vi "SeCrTs-DO Data FGV.vi"(0 "DO Values In":bool[](array[boolean]), 1 "Option":T1(ring)=enum."Start Pattern Mode", 5 "DO Channel Names":string[](array[string]), 9 "Time Stamp In":timestamp, 11 "error in (no error)":errorcluster, 12 "DO Pattern Values In":bool[][](array[boolean])) -> (3 "Expected Completed Time (Pattern)":timestamp, 4 "DO Values Out":bool[](array[boolean]), 6 "All data out":waveform(dbl)[](array[waveform]), 8 "DO Channel Names Out":string[](array[string]), 10 "DO Waveform Out":digitalwaveform[](array[waveform]), 14 "Time Stamp Out":timestamp, 15 "error out":errorcluster)   [LabVIEW 2022 SP3]
uses:
  RT Controls/SeCrTs-FGV Read write.ctl
  <vilib>/Waveform/DTblOps.llb/DTbl Boolean Array to Digital.vi
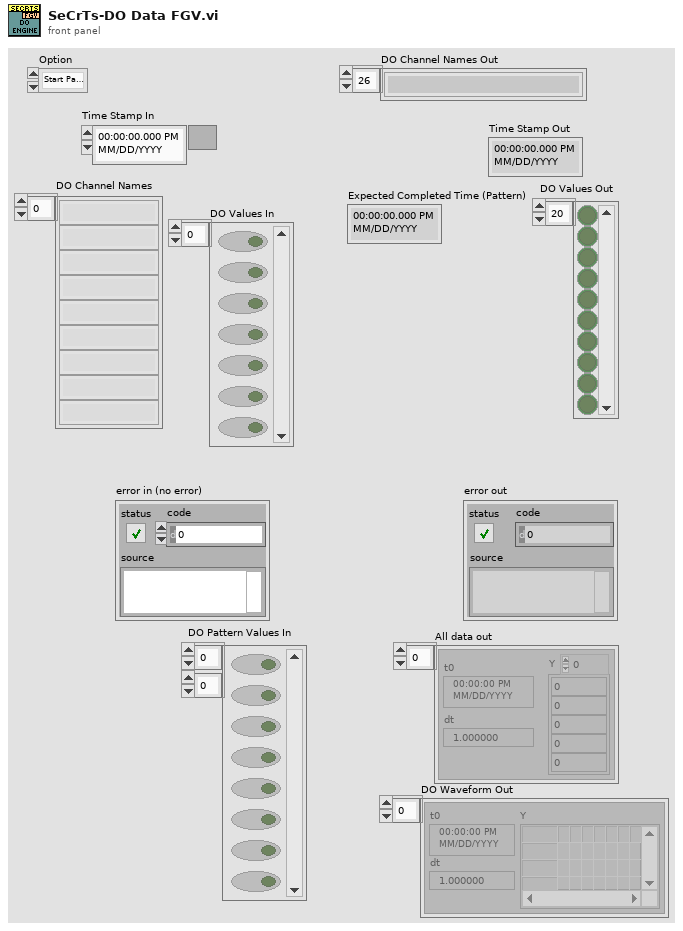
[diagram p1: front panel]
types:
  T1 = enum16{"Init", "Read", "Write 'All'", "Write 'n'", "Write Safe Value", "Write Start Time", "Overwrite Pattern", "Overwrite Pattern with Start", "Append Pattern", "Start Pattern Mode", "Abort Pattern Mode", "Read 1"}
  T2 = typedef "SeCrTs-FGV Read write.ctl" = enum16{"Write", "Read"}
  T3 = cluster{"Samples to Read":i32, "Pattern Mode?":bool, "dt(sec)":dbl, "DO Init Time (Samples)":i32, "dt per Read/Write":dbl, "Write Pointer":i32, "Pattern Size":i32, "Loop Rate (mSec)":i32, "Buffer Size (Samples)":i32, "Sampling rate":dbl, "Max DO Delay Time (samples)":dbl, "Min DO Delay Time (samples)":dbl, "Queue Size":i32, "DO Init Sample Duration (Sec)":dbl}
  T4 = cluster{"Pattern Size":i32, "Write Pointer":i32, "DO Channel Names":string[], "Pattern Mode?":bool, "DO Safe Waveform":waveform(dbl)[], "DO Safe Digital Waveform":digitalwaveform[], "DO Safe Values In":bool[], "dt per Read/Write":dbl}
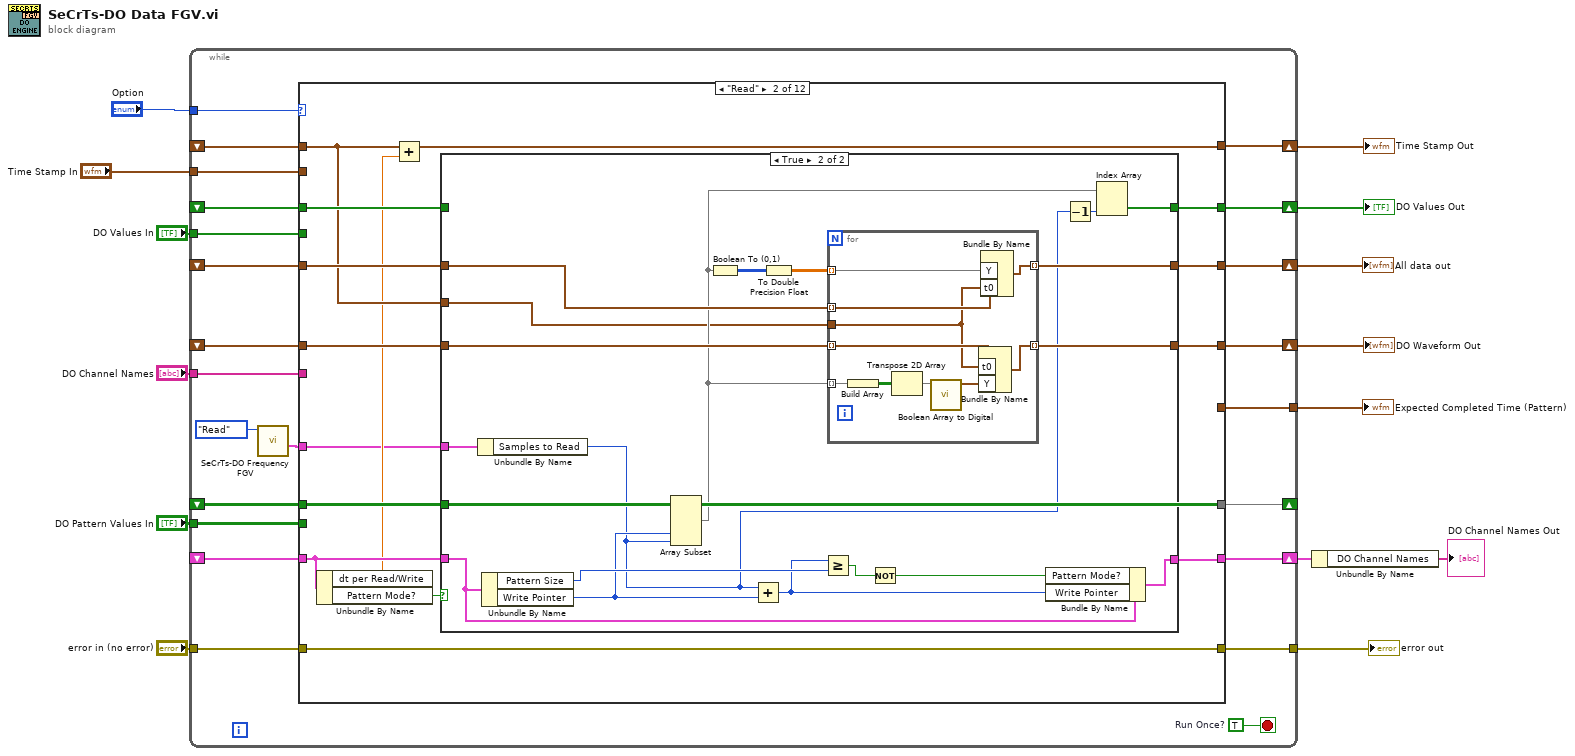
[diagram p0: block diagram]
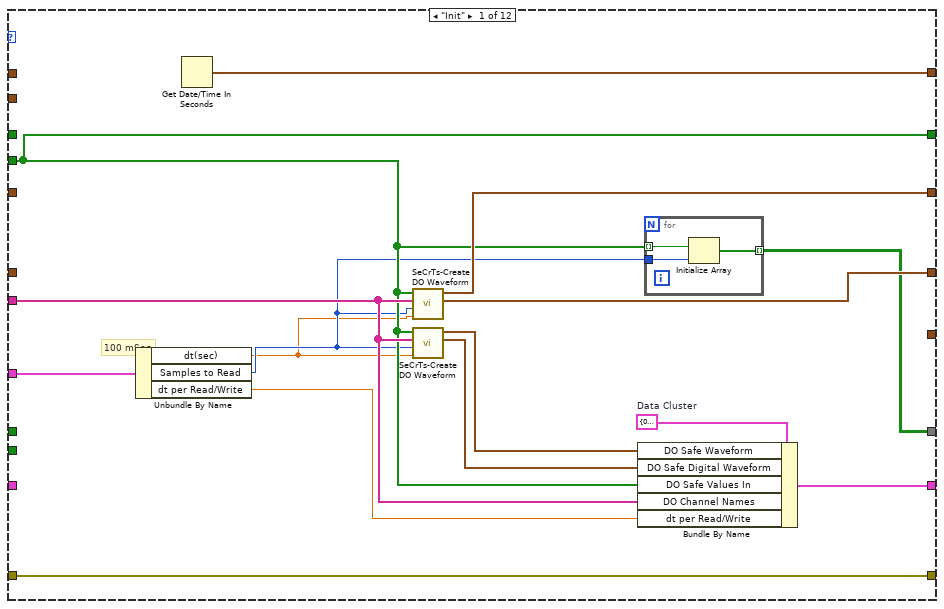
[diagram p2: hidden frame]
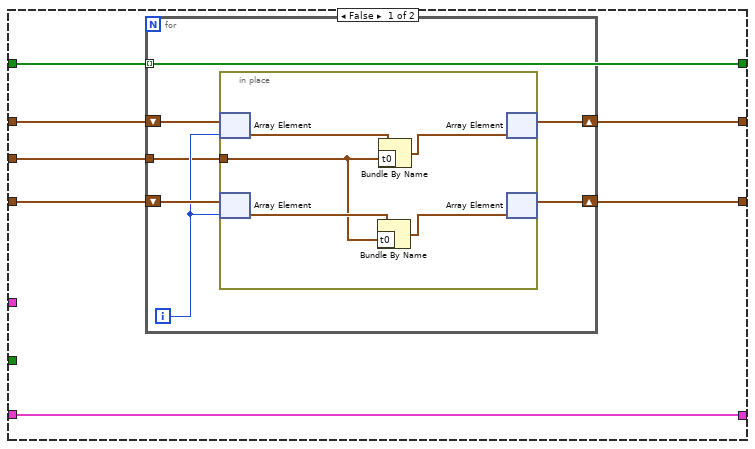
[diagram p3: hidden frame]
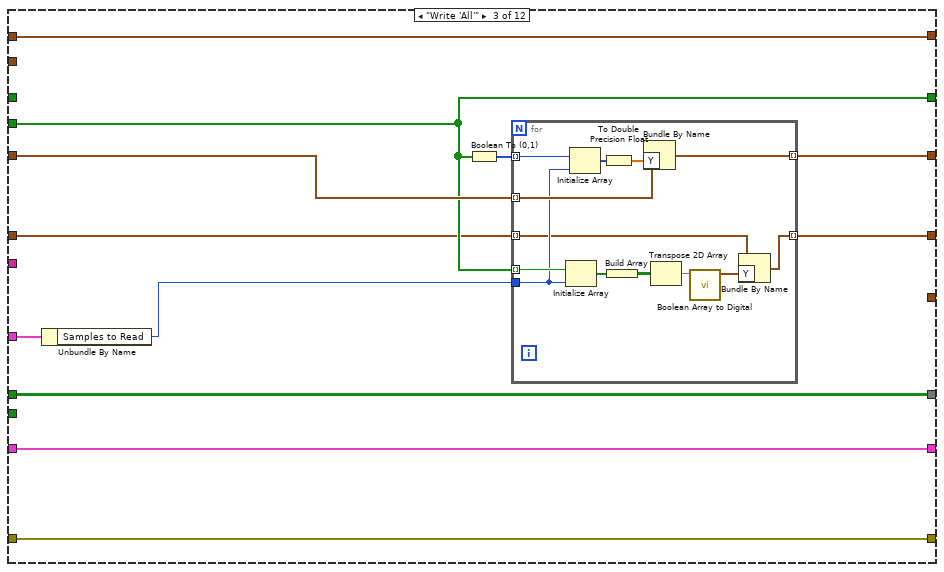
[diagram p4: hidden frame]
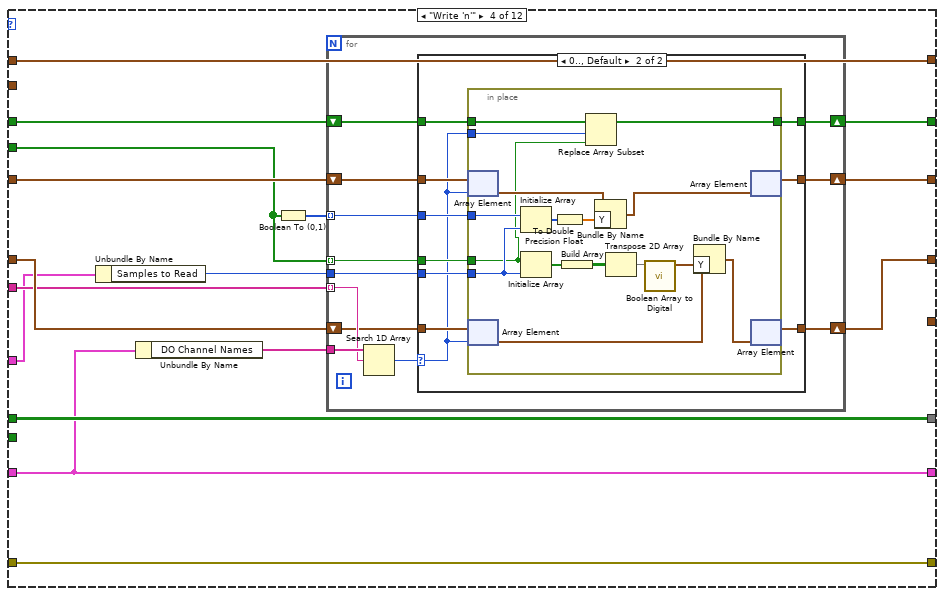
[diagram p5: hidden frame]
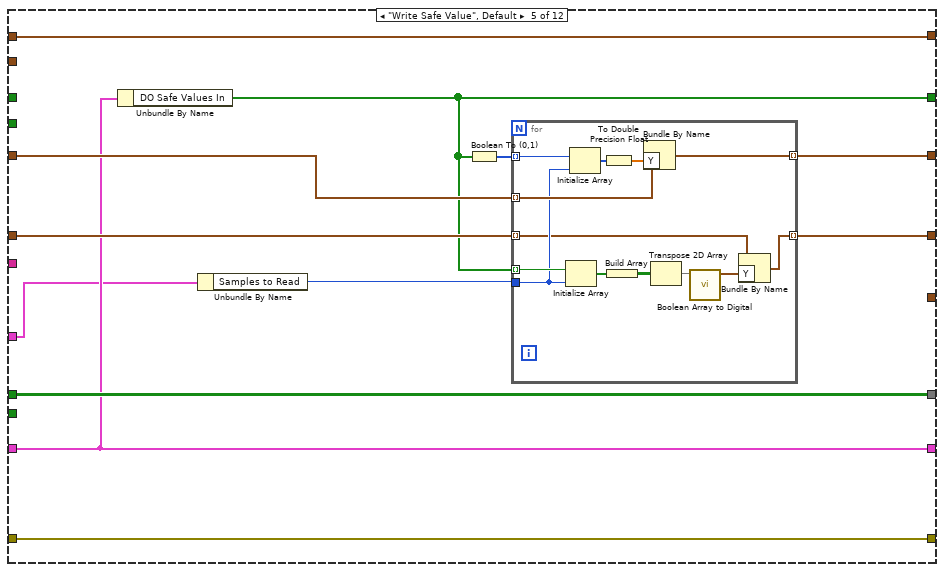
[diagram p7: hidden frame]
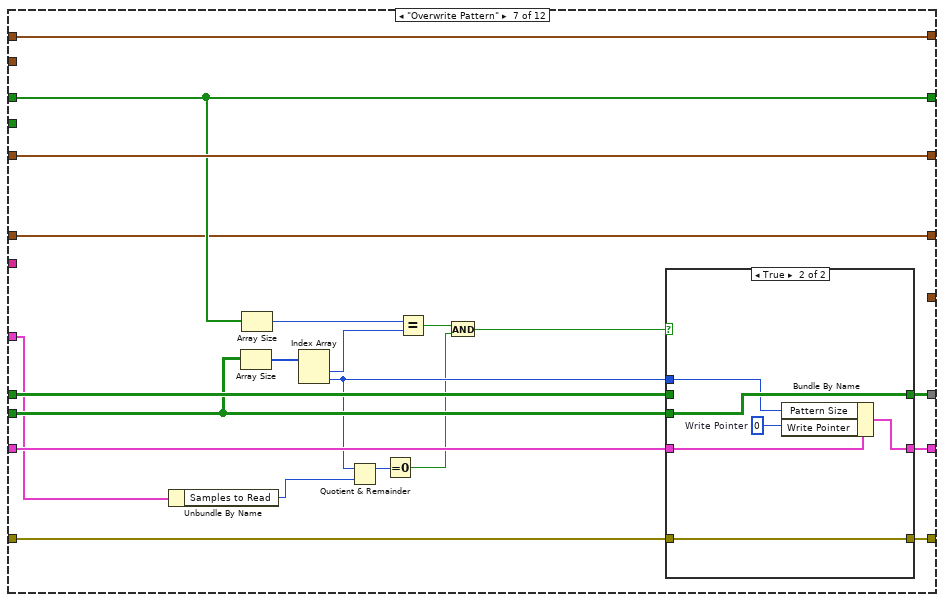
[diagram p9: hidden frame]
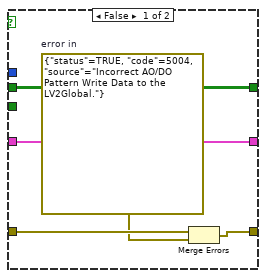
[diagram p10: hidden frame]
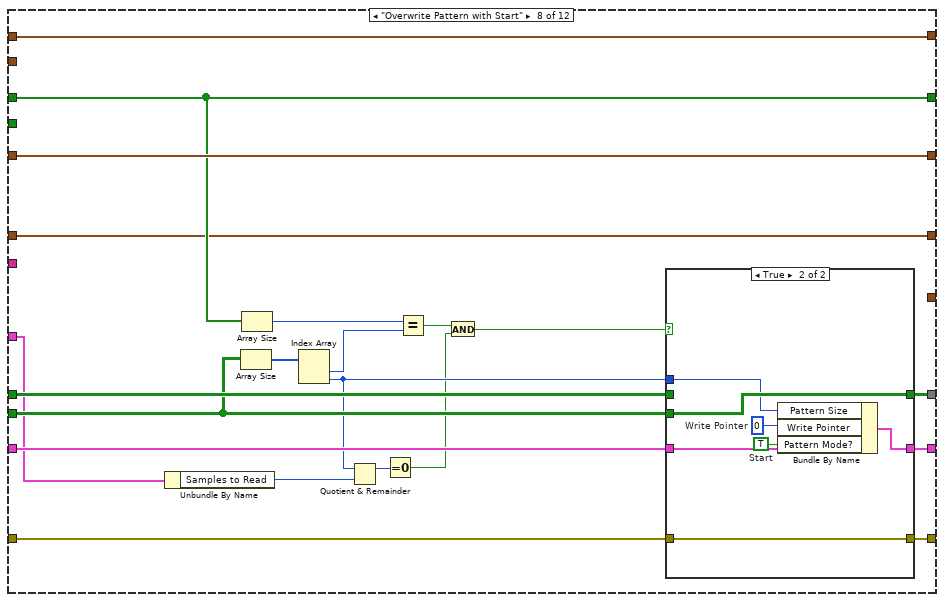
[diagram p11: hidden frame]
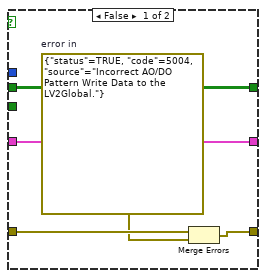
[diagram p12: hidden frame]
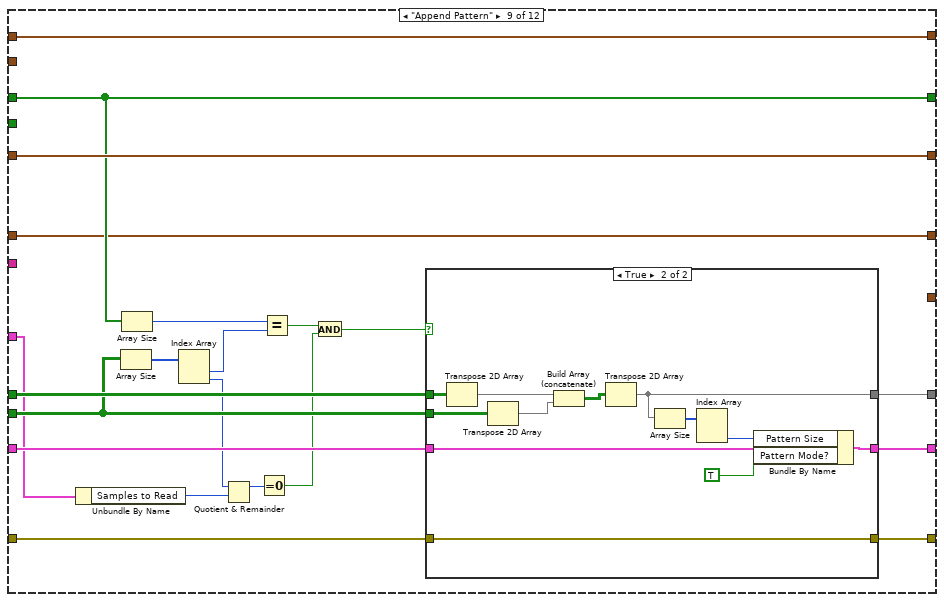
[diagram p13: hidden frame]
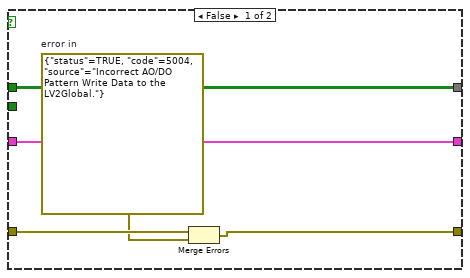
[diagram p14: hidden frame]
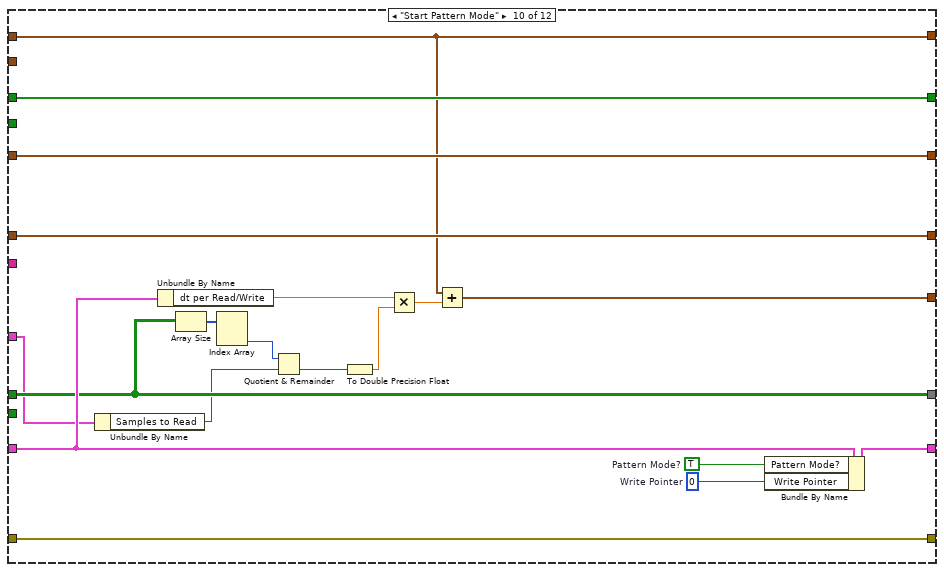
[diagram p15: hidden frame]
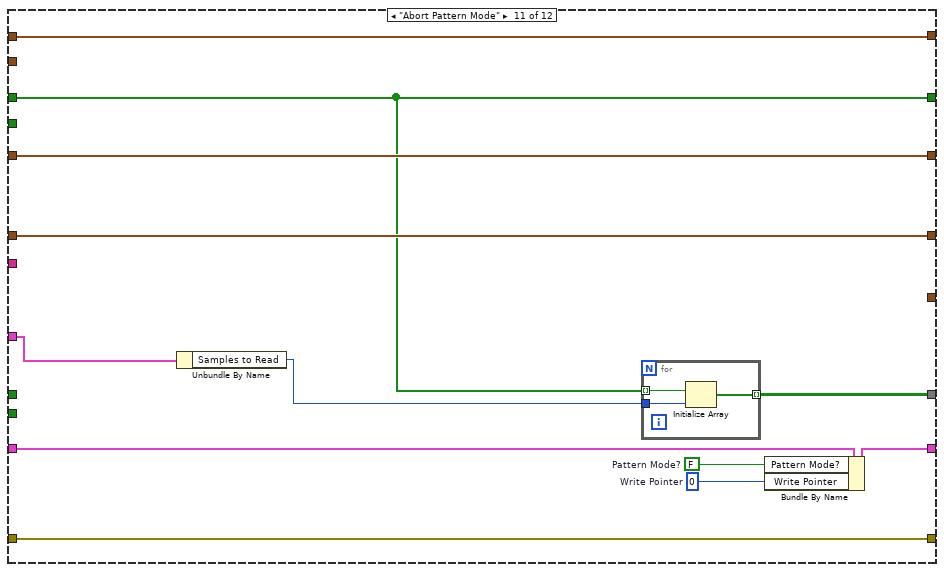
[diagram p16: hidden frame]
diagram:
  n1 = while {
    tunnel: "DO Values In" -> [w35]
    shift-right: [w36] -> w14
    shift-left: _ -> [w34]
    shift-right: [w33] -> w12
    shift-left: _ -> [w32]
    shift-right: [w31] -> w11
    shift-left: _ -> [w30]
    tunnel: "DO Pattern Values In" -> [w27]
    shift-right: [w28] -> _
    shift-left: _ -> [w26]
    shift-right: [w25] -> w2
    shift-left: _ -> [w24]
    tunnel: "error in (no error)" -> [w23]
    tunnel: [w22] -> w7
    tunnel: "DO Channel Names" -> [w21]
    shift-right: [w29] -> w10
    shift-left: _ -> [w20]
    tunnel: "Time Stamp In" -> [w19]
    tunnel: [w18] -> w4
    tunnel: "Option" -> [w17]
    stop <- w37 stop-if-true
    w37 = TRUE  # Run Once?
    n2 = call "SeCrTs-DO Frequency  FGV.vi"("Write/Read"=SeCrTs-FGV_Read_write."Read") -> ("DO Set Frequency (R)"=w15:T3)  [unwired: 9 in, 1 out]
    n3 = case shown="\"Read\"" w17 {
      tunnel: [w43 w61 w125 w146 w203 w232 w251 w283 w316 w354 w359 w376] -> w36
      tunnel: w35 -> [w43 _ w125 w155 _ _ _ _ _ _ _ _]
      tunnel: w34 -> [_ w66 _ w147 _ w232 w251 w283 w316 w354 w359 w376]
      tunnel: [w52 w58 w130 w159 w212 w226 w253 w285 w318 w346 w366 w370] -> w33
      tunnel: w32 -> [_ w59 w130 w159 w212 _ w253 w285 w318 w346 w366 w370]
      tunnel: [w48 w62 w123 w153 w207 w231 w252 w284 w317 w353 w365 w371] -> w31
      tunnel: w30 -> [_ w67 w126 w156 w209 w231 w252 w284 w317 w353 w365 w371]
      tunnel: [w47 w63 w122 w152 w206 w230 w237 w269 w300 w352 w364 w372] -> w29
      tunnel: [w42 w60 w129 w158 w211 w229 w245 w277 w309 w345 w358 w375] -> w28
      tunnel: w27 -> [_ _ _ _ _ _ w243 w275 w307 _ _ _]
      tunnel: w26 -> [_ w60 w129 w158 w211 w229 w244 w276 w308 w345 _ w375]
      tunnel: [w49 w64 w128 w149 w204 w228 w246 w278 w311 w350 w361 w374] -> w25
      tunnel: w24 -> [_ w65 w128 w149 w204 w228 w247 w279 w312 w347 w363 w374]
      tunnel: w23 -> [w50 w70 w127 w157 w210 w227 w242 w274 w306 w351 w362 w373]
      tunnel: [w50 w70 w127 w157 w210 w227 w241 w273 w305 w351 w362 w373] -> w22
      tunnel: w21 -> [w46 _ _ w150 _ _ _ _ _ _ _ _]
      tunnel: w20 -> [_ w68 w121 w151 w205 w230 w237 w269 w300 w352 w364 w372]
      tunnel: w19 -> [_ _ _ _ _ w226 _ _ _ _ _ _]
      tunnel: [_ _ _ _ _ _ _ _ _ w339 _ _] -> w18
      tunnel: w15 -> [w41 w56 w120 w145 w201 _ w233 w265 w299 w336 w355 _]
      frame "Init" {
        w51 = T4 {"Pattern Size"=0, "Write Pointer"=0, "DO Channel Names"=[], "Pattern Mode?"=FALSE, "DO Safe Waveform"=[], "DO Safe Digital Waveform"=[], "DO Safe Values In"=[], "dt per Read/Write"=100.0}  # Data Cluster
        # "100 mSec"
        n4 = Unbundle By Name(w41) -> ("dt(sec)"=w39:dbl, "Samples to Read"=w40:i32, "dt per Read/Write"=w38:dbl)
        n5 = Get Date/Time In Seconds() -> (seconds since 1Jan1904=w52:timestamp)
        n6 = call "SeCrTs-Create DO Waveform.vi"("dt(sec)"=w39, "Size"=w40, "DO Channel Names"=w46, "DO Values In"=w43) -> ("DO Digital Waveform"=w47:digitalwaveform[], "DO Waveform"=w48:waveform(dbl)[])  [unwired: 6 in]
        n7 = call "SeCrTs-Create DO Waveform.vi"("dt(sec)"=w39, "Size"=w40, "DO Channel Names"=w46, "DO Values In"=w43) -> ("DO Digital Waveform"=w44:digitalwaveform[], "DO Waveform"=w45:waveform(dbl)[])  [unwired: 6 in]
        n8 = Bundle By Name(cluster=w51, "DO Safe Waveform"=w45, "DO Safe Digital Waveform"=w44, "DO Safe Values In"=w43, "DO Channel Names"=w46, "dt per Read/Write"=w38) -> (w49:T4)
        n9 = for {
          tunnel: w40 -> [w55]
          tunnel: w43 -> [w54] mode=indexing
          tunnel: [w53] -> w42 mode=indexing
          n10 = Initialize Array(w54, w55) -> (w53:bool[])
        }
      }
      frame "Read" {
        n11 = Unbundle By Name(w65) -> ("dt per Read/Write"=w57:dbl, "Pattern Mode?"=w69:bool)
        n12 = Add(x=w59, y=w57) -> (x+y=w58:timestamp)
        n13 = case shown="True" w69 {
          tunnel: w60 -> [_ w106]
          tunnel: w68 -> [w75 w105]
          tunnel: w67 -> [w76 w102]
          tunnel: w66 -> [w71 _]
          tunnel: w65 -> [w77 w108]
          tunnel: [w77 w107] -> w64
          tunnel: [w73 w104] -> w63
          tunnel: [w74 w103] -> w62
          tunnel: [w71 w100] -> w61
          tunnel: w59 -> [w72 w94]
          tunnel: w56 -> [_ w90]
          frame False {
            n14 = for {
              shift-right: [w80] -> w74
              shift-left: w76 -> [w83]
              shift-right: [w81] -> w73
              shift-left: w75 -> [w82]
              tunnel: w72 -> [w78]
              tunnel: w71 -> [_] mode=indexing
              i -> [w79]
              n15 = in-place {
                in-place-border: w78 -> [w84]
                n16 = in-place-array #1(w83, w79) -> (w88:waveform(dbl))
                n17 = in-place-array #2(w82, w79) -> (w86:digitalwaveform)
                n18 = Bundle By Name(cluster=w86, "t0"=w84) -> (w85:digitalwaveform)
                n19 = Bundle By Name(cluster=w88, "t0"=w84) -> (w87:waveform(dbl))
                n20 = in-place-array #1(w87) -> (w80:waveform(dbl)[])  [unwired: 1 out]
                n21 = in-place-array #2(w85) -> (w81:digitalwaveform[])  [unwired: 1 out]
              }
            }
          }
          frame True {
            n22 = Unbundle By Name(w90) -> ("Samples to Read"=w89:i32)
            n23 = Unbundle By Name(w108) -> ("Pattern Size"=w98:i32, "Write Pointer"=w93:i32)
            n24 = Array Subset(array=w106, index (col)=w93, length (col)=w89) -> (w101:bool[][])  [unwired: 2 in]
            n25 = Boolean To (0,1)(Boolean=w101) -> (0, 1=w96:i16[][])
            n26 = Add(x=w89, y=w93) -> (x+y=w92:i32)
            n27 = To Double Precision Float(number=w96) -> (double precision float=w95:dbl[][])
            n28 = Greater Or Equal?(x=w92, y=w98) -> (x >= y?=w97:bool)
            n29 = for {
              tunnel: [w118] -> w103 mode=indexing
              tunnel: w102 -> [w117] mode=indexing
              tunnel: w101 -> [w111] mode=indexing
              tunnel: [w114] -> w104 mode=indexing
              tunnel: w105 -> [w112] mode=indexing
              tunnel: w95 -> [w110] mode=indexing
              tunnel: w94 -> [w109]
              n30 = Build Array(w111) -> (w116:bool[][])
              n31 = Transpose 2D Array(2D array=w116) -> (transposed array=w113:bool[][])
              n32 = call-poly <vilib>:"Boolean Array to Digital.vi"("boolean array"=w113) -> ("digital data"=w115:digitaldata)  [unwired: 9 in, 1 out]
              n33 = Bundle By Name(cluster=w112, "t0"=w109, "Y"=w115) -> (w114:digitalwaveform)
              n34 = Bundle By Name(cluster=w117, "Y"=w110, "t0"=w109) -> (w118:waveform(dbl))
            }
            n35 = Not(x=w97) -> (.not. x?=w91:bool)
            n36 = Bundle By Name(cluster=w108, "Pattern Mode?"=w91, "Write Pointer"=w92) -> (w107:T4)
            n37 = Decrement(x=w89) -> (x-1=w99:i32)
            n38 = Index Array(array=w101, index (col)=w99) -> (element=w100:bool[])  [unwired: 1 in]
          }
        }
      }
      frame "Write 'All'" {
        n39 = Unbundle By Name(w120) -> ("Samples to Read"=w119:i32)
        n40 = Boolean To (0,1)(Boolean=w125) -> (0, 1=w124:i16[])
        n41 = for {
          tunnel: w124 -> [w142] mode=indexing
          tunnel: [w143] -> w123 mode=indexing
          tunnel: w119 -> [w137]
          tunnel: w126 -> [w139] mode=indexing
          tunnel: w125 -> [w138] mode=indexing
          tunnel: [w133] -> w122 mode=indexing
          tunnel: w121 -> [w131] mode=indexing
          n42 = Initialize Array(w138, w137) -> (w136:bool[])
          n43 = Initialize Array(w142, w137) -> (w141:i16[])
          n44 = To Double Precision Float(number=w141) -> (double precision float=w140:dbl[])
          n45 = Build Array(w136) -> (w135:bool[][])
          n46 = Bundle By Name(cluster=w139, "Y"=w140) -> (w143:waveform(dbl))
          n47 = Transpose 2D Array(2D array=w135) -> (transposed array=w132:bool[][])
          n48 = call-poly <vilib>:"Boolean Array to Digital.vi"("boolean array"=w132) -> ("digital data"=w134:digitaldata)  [unwired: 9 in, 1 out]
          n49 = Bundle By Name(cluster=w131, "Y"=w134) -> (w133:digitalwaveform)
        }
      }
      frame "Write 'n'" {
        n50 = Unbundle By Name(w145) -> ("Samples to Read"=w144:i32)
        n51 = Unbundle By Name(w149) -> ("DO Channel Names"=w148:string[])
        n52 = Boolean To (0,1)(Boolean=w155) -> (0, 1=w154:i16[])
        n53 = for {
          tunnel: w154 -> [w170] mode=indexing
          tunnel: w144 -> [w168]
          tunnel: w155 -> [w169] mode=indexing
          shift-right: [w162] -> w152
          shift-left: w151 -> [w164]
          tunnel: w150 -> [w166] mode=indexing
          tunnel: w148 -> [w167]
          shift-right: [w171] -> w153
          shift-left: w156 -> [w163]
          shift-right: [w160] -> w146
          shift-left: w147 -> [w161]
          n54 = Search 1D Array(1D array=w167, element=w166) -> (index of element=w165:i32)  [unwired: 1 in]
          n55 = case shown="0.., Default" w165 {
            selector: w165 -> [_ w175]
            tunnel: [w174 w179] -> w171
            tunnel: w170 -> [_ w184]
            tunnel: w169 -> [_ w183]
            tunnel: w168 -> [_ w182]
            tunnel: w164 -> [w173 w181]
            tunnel: w163 -> [w174 w180]
            tunnel: [w173 w178] -> w162
            tunnel: w161 -> [w172 w177]
            tunnel: [w172 w176] -> w160
            frame -1 {
            }
            frame 0.., Default {
              n56 = in-place {
                in-place-border: w184 -> [w200]
                in-place-border: w183 -> [w185]
                in-place-border: w182 -> [w197]
                in-place-border: w177 -> [w188]
                in-place-border: [w187] -> w176
                in-place-border: w175 -> [w186]
                n57 = in-place-array #3(w180, w175) -> (w190:waveform(dbl))
                n58 = in-place-array #4(w181, w175) -> (w192:digitalwaveform)
                n59 = Initialize Array(w200, w197) -> (w199:i16[])
                n60 = Initialize Array(w185, w197) -> (w196:bool[])
                n61 = To Double Precision Float(number=w199) -> (double precision float=w198:dbl[])
                n62 = Build Array(w196) -> (w195:bool[][])
                n63 = Replace Array Subset(array=w188, new element=w185, index=w186) -> (w187:bool[])
                n64 = Bundle By Name(cluster=w190, "Y"=w198) -> (w191:waveform(dbl))
                n65 = Transpose 2D Array(2D array=w195) -> (transposed array=w193:bool[][])
                n66 = call-poly <vilib>:"Boolean Array to Digital.vi"("boolean array"=w193) -> ("digital data"=w194:digitaldata)  [unwired: 9 in, 1 out]
                n67 = Bundle By Name(cluster=w192, "Y"=w194) -> (w189:digitalwaveform)
                n68 = in-place-array #3(w191) -> (w179:waveform(dbl)[])  [unwired: 1 out]
                n69 = in-place-array #4(w189) -> (w178:digitalwaveform[])  [unwired: 1 out]
              }
            }
          }
        }
      }
      frame "Write Safe Value", Default {
        n70 = Unbundle By Name(w204) -> ("DO Safe Values In"=w203:bool[])
        n71 = Unbundle By Name(w201) -> ("Samples to Read"=w202:i32)
        n72 = Boolean To (0,1)(Boolean=w203) -> (0, 1=w208:i16[])
        n73 = for {
          tunnel: w208 -> [w224] mode=indexing
          tunnel: [w225] -> w207 mode=indexing
          tunnel: w202 -> [w219]
          tunnel: w209 -> [w221] mode=indexing
          tunnel: w203 -> [w220] mode=indexing
          tunnel: [w215] -> w206 mode=indexing
          tunnel: w205 -> [w213] mode=indexing
          n74 = Initialize Array(w220, w219) -> (w218:bool[])
          n75 = Initialize Array(w224, w219) -> (w223:i16[])
          n76 = To Double Precision Float(number=w223) -> (double precision float=w222:dbl[])
          n77 = Build Array(w218) -> (w217:bool[][])
          n78 = Bundle By Name(cluster=w221, "Y"=w222) -> (w225:waveform(dbl))
          n79 = Transpose 2D Array(2D array=w217) -> (transposed array=w214:bool[][])
          n80 = call-poly <vilib>:"Boolean Array to Digital.vi"("boolean array"=w214) -> ("digital data"=w216:digitaldata)  [unwired: 9 in, 1 out]
          n81 = Bundle By Name(cluster=w213, "Y"=w216) -> (w215:digitalwaveform)
        }
      }
      frame "Write Start Time" {
      }
      frame "Overwrite Pattern" {
        n82 = Unbundle By Name(w233) -> ("Samples to Read"=w234:i32)
        n83 = Array Size(array=w243) -> (size(s)=w250:i32[])
        n84 = Array Size(array=w251) -> (size(s)=w248:i32)
        n85 = Index Array(array=w250) -> (element #1=w249:i32, element #2=w240:i32)  [unwired: 2 in]
        n86 = Quotient & Remainder(x=w240, y=w234) -> (x-y*floor(x/y)=w239:i32)  [unwired: 1 out]
        n87 = Equal To 0?(x=w239) -> (x = 0?=w235:bool)
        n88 = Equal?(x=w248, y=w249) -> (x = y?=w236:bool)
        n89 = And(x=w236, y=w235) -> (x .and. y?=w238:bool)
        n90 = case shown="True" w238 {
          tunnel: w247 -> [w258 w264]
          tunnel: [w258 w263] -> w246
          tunnel: w240 -> [_ w259]
          tunnel: [w257 w261] -> w245
          tunnel: w244 -> [w257 _]
          tunnel: w243 -> [_ w261]
          tunnel: w242 -> [w256 w260]
          tunnel: [w255 w260] -> w241
          frame False {
            w254 = errorcluster {"status"=TRUE, "code"=5004, "source"="Incorrect AO/DO Pattern Write Data to the LV2Global."}  # error in
            n91 = Merge Errors(w256, w254) -> (w255:errorcluster)
          }
          frame True {
            w262 = 0  # Write Pointer
            n92 = Bundle By Name(cluster=w264, "Pattern Size"=w259, "Write Pointer"=w262) -> (w263:T4)
          }
        }
      }
      frame "Overwrite Pattern with Start" {
        n93 = Unbundle By Name(w265) -> ("Samples to Read"=w266:i32)
        n94 = Array Size(array=w275) -> (size(s)=w282:i32[])
        n95 = Array Size(array=w283) -> (size(s)=w280:i32)
        n96 = Index Array(array=w282) -> (element #1=w281:i32, element #2=w272:i32)  [unwired: 2 in]
        n97 = Quotient & Remainder(x=w272, y=w266) -> (x-y*floor(x/y)=w271:i32)  [unwired: 1 out]
        n98 = Equal To 0?(x=w271) -> (x = 0?=w267:bool)
        n99 = Equal?(x=w280, y=w281) -> (x = y?=w268:bool)
        n100 = And(x=w268, y=w267) -> (x .and. y?=w270:bool)
        n101 = case shown="True" w270 {
          tunnel: w279 -> [w290 w297]
          tunnel: [w290 w296] -> w278
          tunnel: w272 -> [_ w291]
          tunnel: [w289 w294] -> w277
          tunnel: w276 -> [w289 _]
          tunnel: w275 -> [_ w294]
          tunnel: w274 -> [w288 w293]
          tunnel: [w287 w293] -> w273
          frame False {
            w286 = errorcluster {"status"=TRUE, "code"=5004, "source"="Incorrect AO/DO Pattern Write Data to the LV2Global."}  # error in
            n102 = Merge Errors(w288, w286) -> (w287:errorcluster)
          }
          frame True {
            w292 = TRUE  # Start
            w295 = 0  # Write Pointer
            n103 = Bundle By Name(cluster=w297, "Pattern Size"=w291, "Write Pointer"=w295, "Pattern Mode?"=w292) -> (w296:T4)
          }
        }
      }
      frame "Append Pattern" {
        n104 = Unbundle By Name(w299) -> ("Samples to Read"=w298:i32)
        n105 = Array Size(array=w307) -> (size(s)=w315:i32[])
        n106 = Array Size(array=w316) -> (size(s)=w313:i32)
        n107 = Index Array(array=w315) -> (element #1=w314:i32, element #2=w303:i32)  [unwired: 2 in]
        n108 = Quotient & Remainder(x=w303, y=w298) -> (x-y*floor(x/y)=w304:i32)  [unwired: 1 out]
        n109 = Equal To 0?(x=w304) -> (x = 0?=w301:bool)
        n110 = Equal?(x=w313, y=w314) -> (x = y?=w310:bool)
        n111 = And(x=w310, y=w301) -> (x .and. y?=w302:bool)
        n112 = case shown="True" w302 {
          tunnel: w312 -> [w323 w335]
          tunnel: [w323 w334] -> w311
          tunnel: [w322 w326] -> w309
          tunnel: w308 -> [w322 w332]
          tunnel: w307 -> [_ w331]
          tunnel: w306 -> [w321 w333]
          tunnel: [w320 w333] -> w305
          frame False {
            w319 = errorcluster {"status"=TRUE, "code"=5004, "source"="Incorrect AO/DO Pattern Write Data to the LV2Global."}  # error in
            n113 = Merge Errors(w321, w319) -> (w320:errorcluster)
          }
          frame True {
            n114 = Transpose 2D Array(2D array=w332) -> (transposed array=w330:bool[][])
            n115 = Transpose 2D Array(2D array=w331) -> (transposed array=w329:bool[][])
            n116 = Build Array (concatenate)(w330, w329) -> (w328:bool[][])
            n117 = Transpose 2D Array(2D array=w328) -> (transposed array=w326:bool[][])
            n118 = Array Size(array=w326) -> (size(s)=w327:i32[])
            n119 = Index Array(array=w327) -> (element #2=w324:i32)  [unwired: 2 in, 1 out]
            n120 = Bundle By Name(cluster=w335, "Pattern Size"=w324, "Pattern Mode?"=TRUE) -> (w334:T4)
          }
        }
      }
      frame "Start Pattern Mode" {
        w348 = 0  # Write Pointer
        w349 = TRUE  # Pattern Mode?
        n121 = Unbundle By Name(w336) -> ("Samples to Read"=w337:i32)
        n122 = Unbundle By Name(w347) -> ("dt per Read/Write"=w342:dbl)
        n123 = Array Size(array=w345) -> (size(s)=w344:i32[])
        n124 = Index Array(array=w344) -> (element #2=w343:i32)  [unwired: 2 in, 1 out]
        n125 = Quotient & Remainder(x=w343, y=w337) -> (floor(x/y)=w338:i32)  [unwired: 1 out]
        n126 = To Double Precision Float(number=w338) -> (double precision float=w340:dbl)
        n127 = Multiply(x=w342, y=w340) -> (x*y=w341:dbl)
        n128 = Add(x=w346, y=w341) -> (x+y=w339:timestamp)
        n129 = Bundle By Name(cluster=w347, "Pattern Mode?"=w349, "Write Pointer"=w348) -> (w350:T4)
      }
      frame "Abort Pattern Mode" {
        w360 = 0  # Write Pointer
        w357 = FALSE  # Pattern Mode?
        n130 = Unbundle By Name(w355) -> ("Samples to Read"=w356:i32)
        n131 = for {
          tunnel: w356 -> [w369]
          tunnel: w359 -> [w368] mode=indexing
          tunnel: [w367] -> w358 mode=indexing
          n132 = Initialize Array(w368, w369) -> (w367:bool[])
        }
        n133 = Bundle By Name(cluster=w363, "Pattern Mode?"=w357, "Write Pointer"=w360) -> (w361:T4)
      }
      frame "Read 1" {
      }
    }
  }
  "error out" <- w7
  "DO Values Out" <- w14
  "Time Stamp Out" <- w12
  "All data out" <- w11
  "DO Waveform Out" <- w10
  "Expected Completed Time (Pattern)" <- w4
  n134 = Unbundle By Name(w2) -> ("DO Channel Names"=→"DO Channel Names Out":string[])
